vi "unormpack.vi"(0 "u03":T1, 1 "u02":T1, 5 "u11":T1, 7 "u12":T1, 9 "u20":T1, 12 "u21":T1, 13 "u30":T1) -> (2 "x/y 7":i32, 3 "x/y 6":i32, 4 "x/y 5":i32, 6 "x/y 4":i32, 8 "x/y 3":i32, 10 "x/y 2":i32, 14 "x/y":i32)   [LabVIEW 2021]
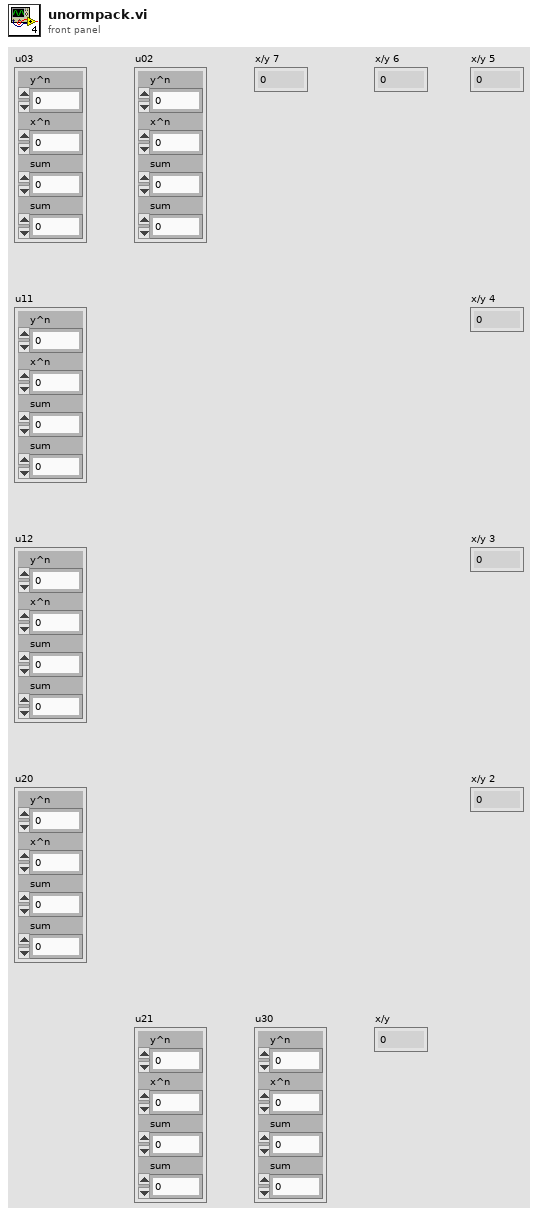
[diagram p1: front panel]
types:
  T1 = cluster{"y^n":dbl, "x^n":dbl, "sum":dbl, "sum":dbl}
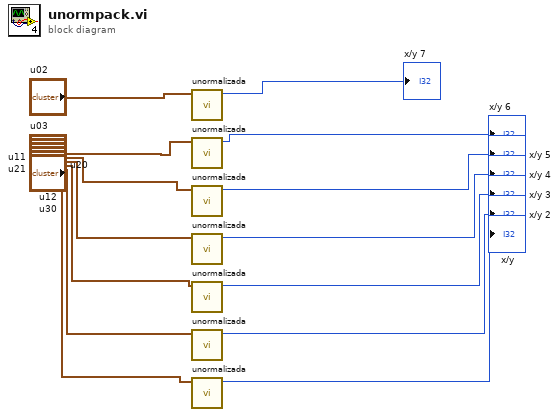
[diagram p0: block diagram]
diagram:
  n1 = call "unormalizada.vi"("upq"="u02") -> ("x/y"=→"x/y 7":i32)  [unwired: 10 in]
  n2 = call "unormalizada.vi"("upq"="u03") -> ("x/y"=→"x/y 6":i32)  [unwired: 10 in]
  n3 = call "unormalizada.vi"("upq"="u11") -> ("x/y"=→"x/y 5":i32)  [unwired: 10 in]
  n4 = call "unormalizada.vi"("upq"="u12") -> ("x/y"=→"x/y 4":i32)  [unwired: 10 in]
  n5 = call "unormalizada.vi"("upq"="u20") -> ("x/y"=→"x/y 3":i32)  [unwired: 10 in]
  n6 = call "unormalizada.vi"("upq"="u21") -> ("x/y"=→"x/y 2":i32)  [unwired: 10 in]
  n7 = call "unormalizada.vi"("upq"="u30") -> ("x/y"=→"x/y":i32)  [unwired: 10 in]
